vi "getZetaFromStart.vi"(8 "Y2":dbl, 9 "X2":dbl, 10 "Y1":dbl, 11 "X1":dbl) -> (1 "dis_*":dbl, 2 "Zeta":dbl)   [LabVIEW 2017]
uses:
  Constant.vi
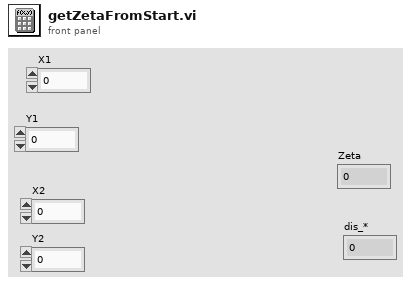
[diagram p1: front panel]
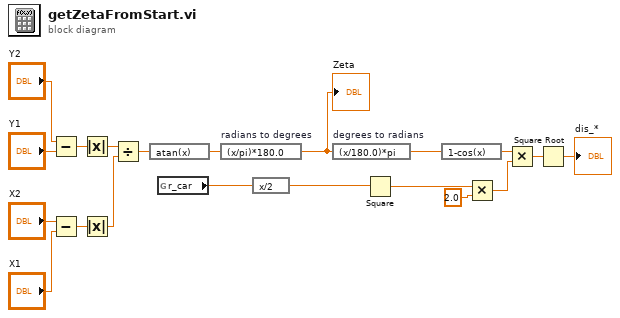
[diagram p0: block diagram]
diagram:
  n1 = Subtract(x="Y2", y="Y1") -> (x-y=w11:dbl)
  n2 = Subtract(x="X2", y="X1") -> (x-y=w14:dbl)
  n3 = Absolute Value(x=w11) -> (abs(x)=w12:dbl)
  n4 = Absolute Value(x=w14) -> (abs(x)=w13:dbl)
  n5 = Divide(x=w12, y=w13) -> (x/y=w16:dbl)
  n6 = expression code="atan(x)"(w16) -> (w15:dbl)
  n7 = global read "Constant.vi" "r_car"() -> (w10:dbl)
  n8 = expression code="(x/pi)*180.0" "radians to degrees"(w15) -> (w2:dbl)
  "Zeta" <- w2
  n9 = expression code="x/2"(w10) -> (w5:dbl)
  n10 = expression code="(x/180.0)*pi" "degrees to radians"(w2) -> (w1:dbl)
  n11 = Square(x=w5) -> (x^2=w9:dbl)
  n12 = expression code="1-cos(x)"(w1) -> (w7:dbl)
  n13 = Multiply(x=w9, y=2.0) -> (x*y=w6:dbl)
  n14 = Multiply(x=w7, y=w6) -> (x*y=w4:dbl)
  n15 = Square Root(x=w4) -> (sqrt(x)=→"dis_*":dbl)
